vi "Average Sectors.vi"(11 "Preanalysis Stage":bool) -> ()   [LabVIEW 2013]
uses:
  Globals/Accumulated Sector Intensity.vi
  <vilib>/rvi/Memory/Memory_Emulation/nirvimemoryFastEmulationFpgaImpl.vi
  <instcachedir>/0/nirvimemoryFastEmulationFpgaImpl_5FBAB50466BC4C939F684F8805638BFC.lvgen/nirvimemoryFastEmulationFpgaImpl_5FBAB50466BC4C939F684F8805638BFC_012.vi
  <vilib>/rvi/DataTransferAndStorage/Container/Common/niFpgaContainerGetUniqueNameForEmu.vi
  <vilib>/rvi/Memory/Memory_Emulation/nirvimemoryFastEmulation.vi
  <vilib>/rvi/Memory/Memory_Emulation/nirvimemoryEmulation.vi
  Globals/Sector Parameter Global.vi
  <vilib>/rvi/FIFO/Fifo_Resource/nirvififoEmulationWriteFpgaImpl.vi
  <vilib>/rvi/DataTransferAndStorage/Container/XNode/niFpgaContainer.xnode
  <vilib>/rvi/FIFO/Fifo_Resource/nirvififoEmulationWrite.vi
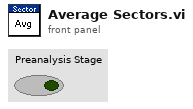
[diagram p1: front panel]
types:
  T1 = cluster{"Accumulated Intensity":fxp<+,20,20>, "Count":fxp<+,12,12>}[]
  T2 = cluster{"Accumulated Intensity":fxp<+,20,20>, "Count":fxp<+,12,12>}
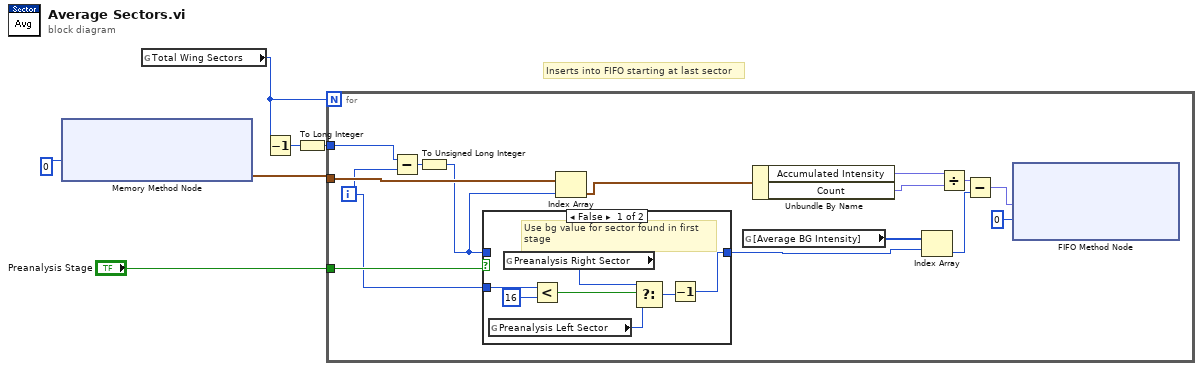
[diagram p0: block diagram]
diagram:
  # "Inserts into FIFO starting at last sector"
  n1 = xnode ("Memory Method Node")("Address"=u32 0) -> ("Data"=w2:T1)  [unwired: 1 in, 1 out]
  n2 = global read "Accumulated Sector Intensity.vi" "Total Wing Sectors"() -> (w4:u8)
  n3 = Decrement(x=w4) -> (x-1=w6:u8)
  n4 = To Long Integer(number=w6) -> (32bit integer=w5:i32)
  n5 = for {
    N: w4 -> [_]
    tunnel: w5 -> [w16]
    tunnel: w2 -> [w14]
    tunnel: "Preanalysis Stage" -> [w10]
    i -> [w7]
    n6 = Subtract(x=w16, y=w7) -> (x-y=w15:i32)
    n7 = To Unsigned Long Integer(number=w15) -> (unsigned 32bit integer=w8:u32)
    n8 = case shown="False" w10 {
      tunnel: [w22 w29] -> w9
      tunnel: w8 -> [_ w29]
      tunnel: w7 -> [w28 _]
      frame False {
        # "Use bg value for sector found in first\nstage"
        n9 = global read "Sector Parameter Global.vi" "Preanalysis Left Sector"() -> (w24:u8)
        n10 = global read "Sector Parameter Global.vi" "Preanalysis Right Sector"() -> (w25:u8)
        n11 = Less?(x=w28, y=16) -> (x < y?=w26:bool)
        n12 = Select(t=w25, s=w26, f=w24) -> (s? t:f=w23:u8)
        n13 = Decrement(x=w23) -> (x-1=w22:u8)
      }
      frame True {
        # "For preanalysis, use the bg\nvalues for the 32 sectors"
      }
    }
    n14 = Index Array(array=w14, index=w8) -> (element=w13:T2)
    n15 = global read "Sector Parameter Global.vi" "[Average BG Intensity]"() -> (w20:u8[])
    n16 = Unbundle By Name(w13) -> ("Accumulated Intensity"=w12:fxp<+,20,20>, "Count"=w11:fxp<+,12,12>)
    n17 = Index Array(array=w20, index=w9) -> (element=w18:u8)
    n18 = Divide(x=w12, y=w11) -> (x/y=w19:fxp<+,8,8>)
    n19 = Subtract(x=w19, y=w18) -> (x-y=w17:fxp<+/-,9,9>)
    n20 = xnode ("FIFO Method Node")("Element"=w17, "Timeout"=0) -> ()  [unwired: 1 in, 2 out]
  }
